vi "Week5_Q1.vi"() -> ()   [LabVIEW 2021, in "LabVIEW Interface for Arduino.lvlib"]
doc: "An example that reads a user selectable analog input pin on the Arduino."
uses:
  <vilib>/LabVIEW Interface for Arduino/LabVIEW Interface for Arduino.lvlib
  <vilib>/LabVIEW Interface for Arduino/Type Defs/Analog Pin.ctl
panel:
  out "Numeric":dbl
  out "Thermometer":dbl(slide) scale=0.0..100.0
  in  "VISA resource":refnum<visa-resource-name>
  in  "Analog Pin":T1
  in  "Stop":bool
  out "Voltage":dbl(knob) scale=0.0..5.0
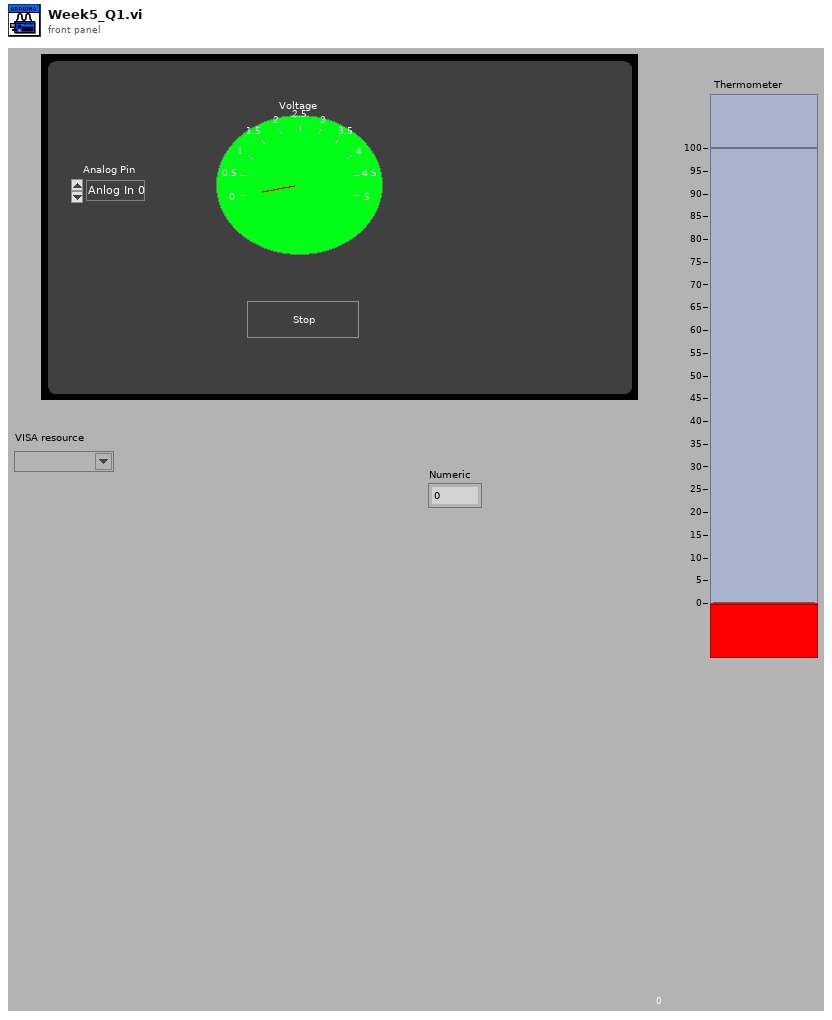
[diagram p1: front panel]
types:
  T1 = typedef "LabVIEW Interface for Arduino.lvlib/Analog Pin.ctl" = enum8{"Anlog In 0", "Anlog In 1", "Anlog In 2", "Anlog In 3", "Anlog In 4", "Anlog In 5"}
  T2 = typedef "LabVIEW Interface for Arduino.lvlib/Arduino Resource.ctl" = cluster{"VISA resource":refnum<visa-resource-name>, "Board Type":T3, "Connection Type":enum8{"USB / Serial"}, "Bytes Per Packet (15)":u8}
  T3 = typedef "LabVIEW Interface for Arduino.lvlib/Board Type.ctl" = enum16{"Uno", "Dimuelanove w/Atmega 328", "Mega 2560"}
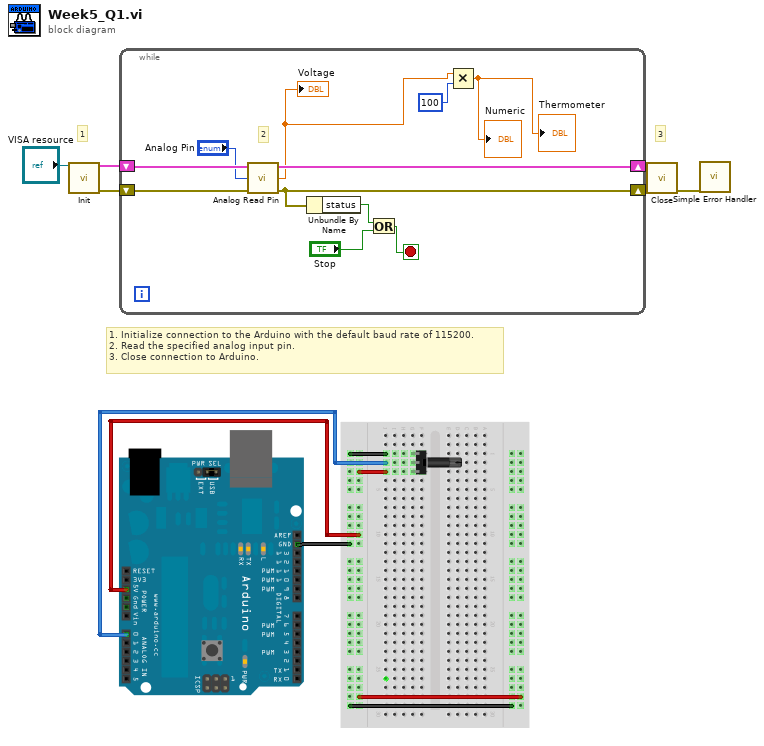
[diagram p0: block diagram]
diagram:
  # "1. Initialize connection to the Arduino with the default baud rate of 115200.\n2. Read the specified analog input pin.\n3. Close connection to Arduino."
  # "3"
  # "1"
  n1 = call <vilib>:"Init.vi"(0:"VISA resource") -> ("Arduino Resource"=w6:T2, "error out"=w3:errorcluster)  [unwired: 17 in]
  n2 = while {
    shift-right: [w17] -> w5
    shift-left: w6 -> [w12]
    shift-right: [w16] -> w4
    shift-left: w3 -> [w11]
    stop <- w15 stop-if-true
    # "2"
    n3 = call <vilib>:"Analog Read Pin.vi"("Arduino Resource"=w12, "Analog Input Pin (0)"="Analog Pin", "error in"=w11) -> ("Arduino Resource"=w17:T2, "Voltage"=w9:dbl, "error out"=w16:errorcluster)  [unwired: 10 in]
    "Voltage" <- w9
    n4 = Unbundle By Name(w16) -> ("status"=w14:bool)
    n5 = Or(x=w14, y="Stop") -> (x .or. y?=w15:bool)
    n6 = Multiply(x=w9, y=100) -> (x*y=→"Thermometer" →"Numeric":dbl)
  }
  n7 = call <vilib>:"Close.vi"("Arduino Resource"=w5, "error in"=w4) -> ("error out"=w2:errorcluster)  [unwired: 13 in]
  n8 = call <vilib>:"Simple Error Handler.vi"("error in (no error)"=w2) -> ()  [unwired: 4 in, 5 out]
